vi "Queued State Machine.vi"() -> ()   [LabVIEW 2010]
doc: "이 VI는 큐 기반 상태 머신의 템플릿입니다. 프로세스 1 및 프로세스 2를 사용자의 상태로 대체하십시오. 더 많은 프로세스를 추가하려면, 타입 정의된 열거형 상수를 수정하십시오. 열거형 순서는 클러스터 순서와 일치해야 합니다."
uses:
  Queued State Enum.ctl
panel:
  in  "메뉴":T1
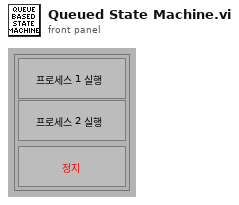
[diagram p1: front panel]
types:
  T1 = cluster{"Process 1":bool, "Process 2":bool, "stop":bool}
  T2 = typedef "Queued State Enum.ctl" = enum32{"유휴", "프로세스 1", "프로세스 2", "정지"}
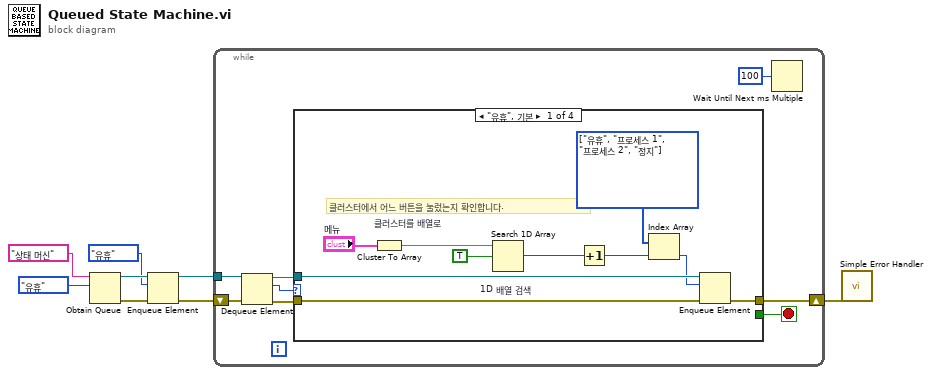
[diagram p0: block diagram]
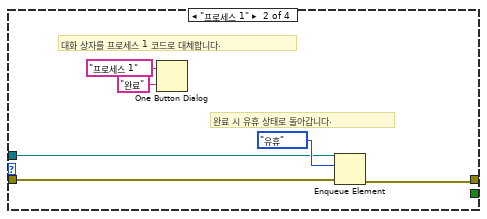
[diagram p2: hidden frame]
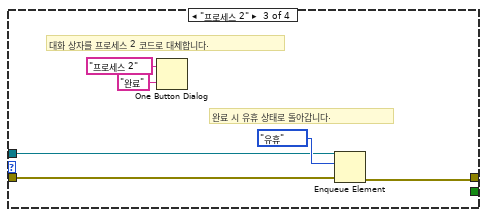
[diagram p3: hidden frame]
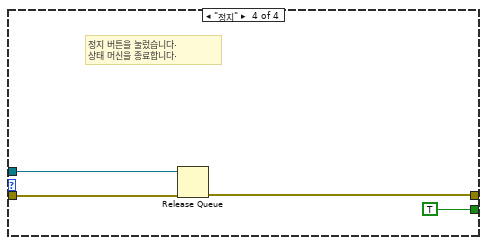
[diagram p4: hidden frame]
diagram:
  n1 = Obtain Queue(name (unnamed)="상태 머신", element data type=Queued_State_Enum."유휴" ("Enum")) -> (queue out=w6:refnum<queue>, error out=w7:errorcluster)  [unwired: 3 in, 1 out]
  n2 = Enqueue Element(queue=w6, element=Queued_State_Enum."유휴" ("Enum"), error in (no error)=w7) -> (queue out=w4:refnum<queue>, error out=w5:errorcluster)  [unwired: 2 out]
  n3 = while {
    tunnel: w4 -> [w11]
    shift-right: [w14] -> w1
    shift-left: w5 -> [w13]
    stop <- w16 stop-if-true
    n4 = Dequeue Element(queue=w11, error in (no error)=w13) -> (queue out=w10:refnum<queue>, element=w9:T2, error out=w12:errorcluster)  [unwired: 2 out]
    n5 = case shown="\"유휴\", 기본" w9 {
      tunnel: [_ _ _ TRUE] -> w16
      tunnel: w12 -> [w22 w30 w36 w41]
      tunnel: w10 -> [w21 w27 w33 w40]
      tunnel: [w20 w29 w35 w39] -> w14
      frame "유휴", Default {
        w18 = T2[] [enum."유휴", enum."프로세스 1", enum."프로세스 2", enum."정지"] items=["유휴", "프로세스 1", "프로세스 2", "정지"]
        # "클러스터에서 어느 버튼을 눌렀는지 확인합니다."
        n6 = Cluster To Array "클러스터를 배열로"(cluster="메뉴") -> (array=w25:bool[])
        n7 = Search 1D Array "1D 배열 검색"(1D array=w25, element=TRUE) -> (index of element=w23:i32)  [unwired: 1 in]
        n8 = Increment(x=w23) -> (x+1=w19:i32)
        n9 = Index Array(array=w18, index=w19) -> (element=w17:T2)
        n10 = Enqueue Element(queue=w21, element=w17, error in (no error)=w22) -> (error out=w20:errorcluster)  [unwired: 3 out]
      }
      frame "프로세스 1" {
        # "완료 시 유휴 상태로 돌아갑니다."
        # "대화 상자를 프로세스 1 코드로 대체합니다."
        n11 = One Button Dialog(message="프로세스 1", button name ("OK")="완료") -> ()  [unwired: 1 out]
        n12 = Enqueue Element(queue=w27, element=Queued_State_Enum."유휴" ("Enum"), error in (no error)=w30) -> (error out=w29:errorcluster)  [unwired: 3 out]
      }
      frame "프로세스 2" {
        # "완료 시 유휴 상태로 돌아갑니다."
        # "대화 상자를 프로세스 2 코드로 대체합니다."
        n13 = One Button Dialog(message="프로세스 2", button name ("OK")="완료") -> ()  [unwired: 1 out]
        n14 = Enqueue Element(queue=w33, element=Queued_State_Enum."유휴" ("Enum"), error in (no error)=w36) -> (error out=w35:errorcluster)  [unwired: 3 out]
      }
      frame "정지" {
        # "정지 버튼을 눌렀습니다.\n상태 머신을 종료합니다."
        n15 = Release Queue(queue=w40, error in (no error)=w41) -> (error out=w39:errorcluster)  [unwired: 1 in, 2 out]
      }
    }
    n16 = Wait Until Next ms Multiple(millisecond multiple=u32 100) -> ()  [unwired: 1 out]
  }
  n17 = call <vilib>:"Simple Error Handler.vi"("error in (no error)"=w1) -> ()  [unwired: 1 in, 8 out]
